vi "Read Control Label.vi"(8 "error in (no error)":errorcluster, 11 "ValueChangeMsg in":refnum<class "ValueChangeMsg.lvclass">) -> (0 "error out":errorcluster, 2 "Control Label":string, 3 "ValueChangeMsg out":refnum<class "ValueChangeMsg.lvclass">)   [LabVIEW 2015, in "ActorEvents.lvlib" / "ValueChangeMsg.lvclass"]
uses:
  ValueChangeMsg.lvclass
  ValueChangeMsg.lvclass/ValueChangeMsg.ctl
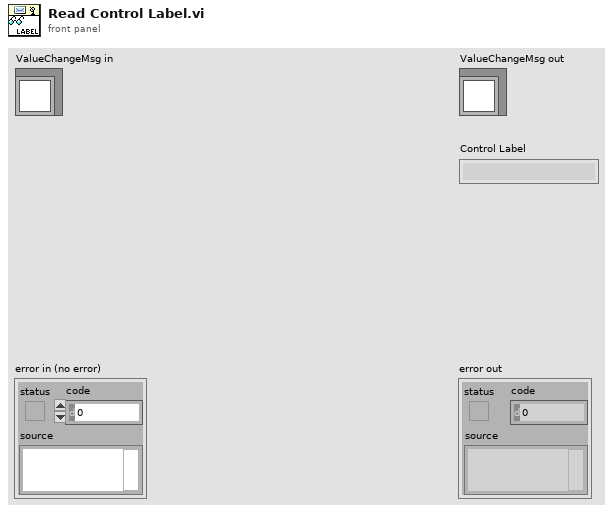
[diagram p1: front panel]
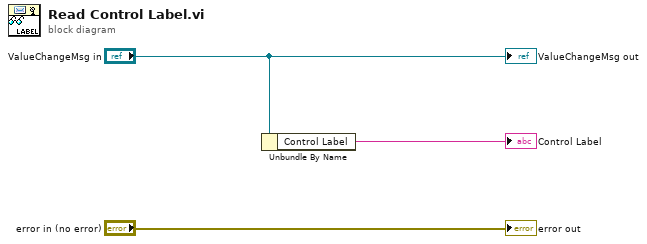
[diagram p0: block diagram]
diagram:
  n1 = Unbundle By Name("ValueChangeMsg in") -> ("Control Label"=→"Control Label":string)
  "error out" <- "error in (no error)"
  "ValueChangeMsg out" <- "ValueChangeMsg in"
